vi "Handle setAllData.vi"(8 "error in (no error)":errorcluster, 10 "AllData":variant, 11 "Inst.Krohn-Hite-7008 in":refnum<class "Inst.Krohn-Hite-7008.lvclass">) -> (0 "error out":errorcluster, 3 "Inst.Krohn-Hite-7008 out":refnum<class "Inst.Krohn-Hite-7008.lvclass">)   [LabVIEW 2019, in "Inst.Krohn-Hite-7008.lvclass"]
doc: "Override to handle \"getAll\" or \"getAllData\" commands for <b>your</b> Instrument"
uses:
  Inst.Krohn-Hite-7008.lvclass
  Inst.Krohn-Hite-7008.lvclass/Inst.Krohn-Hite-7008.ctl
  c49c3efa-452e-49ef-a203-a6ff3341f9e6.vi
  c49c3efa-452e-49ef-a203-a6ff3341f9e6.vi/613b53cc-b559-4394-bfe6-2121b1403f43.vi
  c49c3efa-452e-49ef-a203-a6ff3341f9e6.vi/bee43539-e071-456e-920d-0ce515082382.vi
  <vilib>/Utility/Data Type/Get Type Information.vi
  <vilib>/JDP Science/JSONtext/JSON text to Variant.vi
  <vilib>/JDP Science/JSONtext/LVClass Serializer/JSONtext LVClass Serializer.lvclass
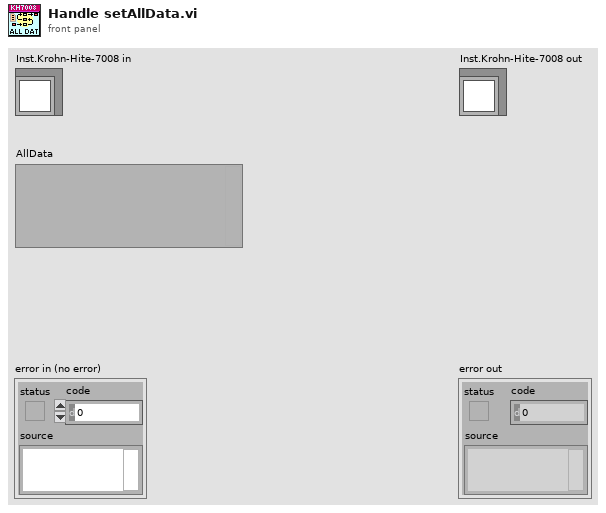
[diagram p1: front panel]
types:
  T1 = typedef "KH7008.lvlib/allChannelProperties--Array.ctl" = T2[]
  T2 = typedef "KH7008.lvlib/channelProperties--Cluster.ctl" = cluster{"channel":T3, "gain":T4, "input":T5, "shunt":T6, "couple":T7, "filter":T8}
  T3 = typedef "KH7008.lvlib/channel--numeric.ctl" = u16
  T4 = typedef "KH7008.lvlib/gain--enum.ctl" = enum16{"1", "10", "100", "1000"}
  T5 = typedef "KH7008.lvlib/input--enum.ctl" = enum16{"OFF", "SE+", "SE-", "DIFF"}
  T6 = typedef "KH7008.lvlib/shunt--enum.ctl" = enum16{"Open", "50", "500", "5k", "50k", "10M"}
  T7 = typedef "KH7008.lvlib/couple--enum.ctl" = enum16{"AC", "DC"}
  T8 = typedef "KH7008.lvlib/filter--enum.ctl" = enum16{"OFF", "ON"}
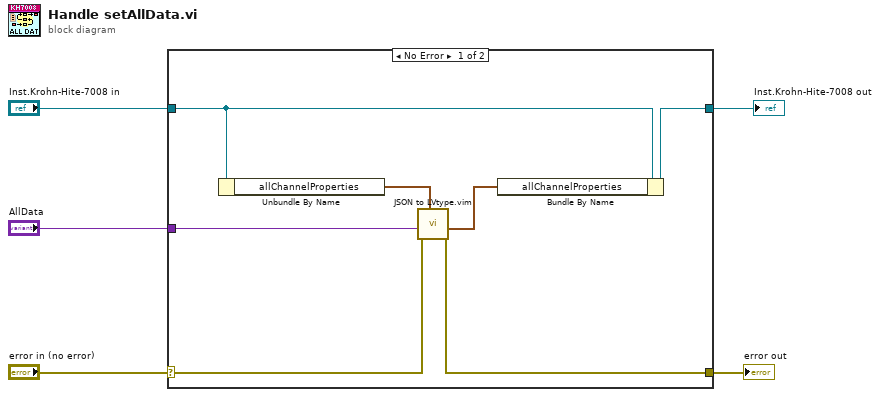
[diagram p0: block diagram]
diagram:
  n1 = case shown="No Error" "error in (no error)" {
    selector: "error in (no error)" -> [w8 w14]
    tunnel: [w7 w14] -> w3
    tunnel: [w12 w13] -> w4
    tunnel: "Inst.Krohn-Hite-7008 in" -> [w11 w13]
    tunnel: "AllData" -> [w9 _]
    frame No Error {
      n2 = Unbundle By Name(w11) -> ("allChannelProperties"=w10:T1)
      n3 = call "JSON to LVtype.vim"("type"=w10, "error in (no error)"=w8, "JSON Data in"=w9) -> ("error out"=w7:errorcluster, "Data out"=w6:T2[])  [unwired: 7 in]
      n4 = Bundle By Name(cluster=w11, "allChannelProperties"=w6) -> (w12:refnum<class "Inst.Krohn-Hite-7008.lvclass">)
    }
    frame Error {
    }
  }
  "error out" <- w3
  "Inst.Krohn-Hite-7008 out" <- w4
